vi "Pre Launch Init.vi"(11 "ZenGage v3.0 UI in":refnum<class "ZenGage v3.0 UI.lvclass">) -> (0 "error out":errorcluster, 3 "ZenGage v3.0 UI out":refnum<class "ZenGage v3.0 UI.lvclass">)   [LabVIEW 2019, in "ZenGage v3.0 UI.lvclass"]
doc: "(<B>Filename</B>: Actor Framework.lvlib:Actor.lvclass:Pre Launch Init.vi)\n\nDefines behavior that occurs after the Launch Nested Actor method is invoked but before the actor's Actor Core method begins running.\n\nBy default, this method does nothing. A descendant class may override it to define behavior."
uses:
  ZenGage v3.0 UI.lvclass
  <vilib>/vision/Image Controls.llb/IMAQ Image.ctl
  Type Definitions/User Events UI/LoadingBar_General_UI.ctl
  Type Definitions/User Events UI/Stop slave cluster.ctl
  Type Definitions/User Events UI/Optics diagnostics cluster.ctl
  Type Definitions/JSON Read/Data initialization.ctl
  Type Definitions/JSON Read/Post select init.ctl
  Type Definitions/Diagnostics/Trigger sensor.ctl
  Common/Controls/Pop-up Input.ctl
  Type Definitions/Inspection/Result Cluster.ctl
  <vilib>/ActorFramework/Actor/Actor.lvclass
  Type Definitions/JSON Read/UI JSON read cluster.ctl
  Type Definitions/General/JSONRead.ctl
  Type Definitions/Inspection/Inspection Cluster.ctl
  Type Definitions/Diagnostics/Diagnostics(Cluster).ctl
  Type Definitions/Edit tolerance settings/Rack Selection.ctl
  <vilib>/Utility/miscctls.llb/LVPoint32TypeDef.ctl
  Type Definitions/Edit tolerance settings/Edit Tolerance Input.ctl
  Type Definitions/Edit tolerance settings/Edit Tolerance Overall Cluster.ctl
  Type Definitions/Controls and Indicators/Inspection control references.ctl
  Type Definitions/Controls and Indicators/Diagnostics control referencs.ctl
  Type Definitions/Controls and Indicators/EDL control references.ctl
  Type Definitions/Controls and Indicators/Controls and Indicators Cluster.ctl
  Type Definitions/General/UI States(UI button enable disable).ctl
  Type Definitions/General/UIDataCluster.ctl
  Type Definitions/Controls and Indicators/General_Control references.ctl
  Type Definitions/General/Master sample references.ctl
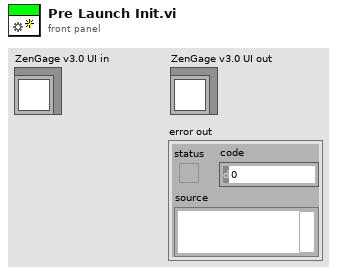
[diagram p1: front panel]
types:
  T1 = cluster{"Master sample message":string, "Part message":string}
  T2 = typedef "ZenGage v3.0 UI.lvclass/Result Cluster.ctl" = cluster{"Rack Id":u64, "Measurement Values Array ":dbl[], "Images_Array_in":T3[], "ResultPF":bool, "Production count details":cluster{"Total Count":dbl, "Total Pass":dbl, "Total Fail":dbl}, "Control Pass Fail":bool[], "ReelCount Details":cluster{"Reel Count":dbl, "Reel Pass":dbl, "Reel Fail":dbl}, "Specification Pass Fail":bool[], "SpecificationFail":bool}
  T3 = typedef "IMAQ Image.ctl" = refnum<image>
  T4 = typedef "UIDataCluster.ctl" = cluster{"JSONRead":T5, "Inspection":T7, "Diagnostics":T8, "EditToleranceSettings":T9, "ControlsIndicators":T13, "AdditionalFeatures":cluster{"Cp Cpk details":cluster{"CpCpkData":string[][], "Cp Cpk popup":refnum<vi>}, "Popup":cluster{"Restore main tab":string, "Popup data":cluster{"Loading bar data":cluster{"Open?":bool, "Display string":string}, "Pop-up":T19}}, "DynamicImageHandling":cluster{"Image update":cluster{"Rack Id":i32, "Update image":bool[]}[], "RBCIA":cluster{"Rack Id":u8, "Imaging view names":string[]}[], "ISIM":u8[], "Camera labels list":string[], "Enable DIH?":bool, "Init DIH params?":bool}, "PageHandling":cluster{"Previous State":T20, "Current state":string, "Previous control access state":string}, "Core":cluster{"Current VI Reference":refnum<vi>, "Close Panel on Exit?":bool}, "SlaveLoopData":cluster{"EnableShortKeyPress":bool, "Point32":T12}, "Chosen event reason":string, "Master sample validation":cluster{"Master sample general message":string, "Master sample part message":string}, "Fail Ignore Count Reversal":cluster{"Production ignored count":u64, "Reel ignored count":u64}}}
  T5 = typedef "ZenGage v3.0 UI.lvclass/JSONRead.ctl" = cluster{"ConfigurationFilePaths":cluster{"Default JSON Path in":path, "Rack Controller Override JSON file path in":path, "Algorithm Overrride JSON file path in ":path}, "ConfigurationVariants":cluster{"Default JSON \nVariant":variant, "Algorithm Override\nJSON Variant":variant, "Rack Controller Override\nJSON Variant":variant}, "ConfigurationCluster":T6}
  T6 = typedef "ZenGage v3.0 UI.lvclass/UI JSON read cluster.ctl" = cluster{"UIParameters":cluster{"SpecificationVersion":string, "Title":string, "NumberOfImagesToBeDisplayed":dbl, "ImageCountWindow":dbl, "FontName":string, "FontSize":dbl, "CustomerLogoFilePath":string, "ZentronLogoFilePath":string, "CompatibleSoftwareVersions":string[], "CameraLabelMapping":cluster{"CameraName":string, "ImageLabel":string}[], "ImageIndicatorLayouts":cluster{"NumberOfImageIndicators":dbl, "ImageSpecificData":cluster{"Width":dbl, "Left":dbl, "Top":dbl, "ImagePercentage":cluster{"Height":dbl, "Widthcorrection":i64, "Heightcorrection":i64, "Leftcorrection":dbl, "Topcorrection":dbl}, "StringPercentage":cluster{"Height":dbl, "Widthcorrection":i64, "Heightcorrection":dbl, "Leftcorrection":dbl, "Topcorrection":dbl}}[]}[], "SoftwareButtonLabels":cluster{"SelectLabel":string, "RunLabel":string, "PauseLabel":string, "StopLabel":string}, "DiagnosticsParameters":cluster{"CameraOpticsDiagnostics":cluster{"Label":string, "CameraLabelsList":cluster{"CameraName":string, "ImageLabel":string}[]}, "ArduinoDiagnostics":cluster{"Label":string}, "MotorDiagnostics":cluster{"Label":string}, "ReelerMotor":cluster{"Label":string}, "TowerLampDiagnostics":cluster{"Label":string}, "TriggerSensor":cluster{"Label":string, "SensorsList":cluster{"SensorName":string, "LabelName":string}[]}, "HardwareButtonDiagnostics":cluster{"Label":string}, "MasterSampleDiagnostics":cluster{"Label":string}}, "DieIdParameters":cluster{"DefaultDieId":string, "DieIdsList":string[]}, "EventReasonsList":cluster{"Pause":string[], "Stop":string[], "FailPause":string[], "Ignored":string[], "DefaultEventReason":string}, "StampingMachineIds":string[], "ErrorPopupStrings":cluster{"ErrorCode":string, "ErrorString":string}[]}}
  T7 = typedef "ZenGage v3.0 UI.lvclass/Inspection Cluster.ctl" = cluster{"Inspection After Stop":bool, "IsPaused":bool, "Camera Names":string[], "Fail Array":bool[], "Reel Number":u32, "Image details_init":cluster{"Mapped view names":string[], "Camera image map array":i32[], "Camera names":string[]}[], "LSL":string[], "USL":string[], "Max limits":cluster{"Production max":u64, "Reel max":u64}, "parts List":string[], "#Racks":u8, "MeasurementNames":string[], "Reel complete":bool, "Fail event reason list":string[]}
  T8 = typedef "ZenGage v3.0 UI.lvclass/Diagnostics(Cluster).ctl" = cluster{"Selection Done?":bool, "Diagnostics details":cluster{"Diagnostics names":cluster{"Main diagnostics":string[], "Sub diagnostics names":cluster{"Camera optics":string[], "Trigger sensor":string[]}}, "Diagnostics labels":cluster{"Main diagnostics":string[], "Sub diagnostics names":cluster{"Camera optics":string[], "Trigger sensor":string[]}}}, "DiagnosticsFeatures":cluster{"ArduinoDiagnostics":bool, "MotorDiagnostics":bool, "CameraOpticsDiagnostics":bool, "ReelerMotor":bool, "HardwareButtonDiagnostics":bool, "TriggerSensor":bool, "TowerLampDiagnostics":bool, "MasterSampleDiagnostics":bool}, "SelectedDiagnostics":string}
  T9 = typedef "ZenGage v3.0 UI.lvclass/Edit Tolerance Overall Cluster.ctl" = cluster{"Input ListBox":T10, "Saved?":bool, "IsETLSelected":bool, "IsPartSelected":bool}
  T10 = typedef "ZenGage v3.0 UI.lvclass/Edit Tolerance Input.ctl" = cluster{"Measurement Values":string[][], "Cluster of Limits":cluster{"LSL":dbl, "USL":dbl, "LCL":dbl, "UCL":dbl}, "Rack Selection":T11, "M and N Array":cluster{"M1":u64, "M2":u64, "N1":u64, "N2":u64}[], "Ticked Measurement Index":u32[], "Measurements Enabled":bool[], "Current Active Position":T12, "Current ticked measurement":dbl}
  T11 = typedef "ZenGage v3.0 UI.lvclass/Rack Selection.ctl" = enum16{"Both Racks", "Rack 2", "Rack 1"}
  T12 = typedef "LVPoint32TypeDef.ctl" = cluster{"Horizontal":i32, "Vertical":i32}
  T13 = typedef "ZenGage v3.0 UI.lvclass/Controls and Indicators Cluster.ctl" = cluster{"General":T14, "Inspection":T15, "Diagnostics":T16, "Edit Tolerance Limits":T17, "Master sample":T18}
  T14 = typedef "ZenGage v3.0 UI.lvclass/General_Control references.ctl" = cluster{"Main Tab":refnum<vi>, "Inspection SubPanel_Inspection":refnum<vi>, "Zen Logo_Inspection":refnum<vi>, "SoftwareExit":refnum<vi>, "Loading Bar VI Ref":refnum<vi>, "Right Pane Tab":refnum<vi>, "Image Reference array":refnum<vi>[], "Command tab":refnum<vi>, "Inspection subTab control ref":refnum<vi>, "SelectionCluster":cluster{"ok":refnum<vi>, "confirm":refnum<vi>, "reset":refnum<vi>, "change":refnum<vi>, "TOTAL COUNT":refnum<vi>, "REEL COUNT":refnum<vi>, "PART NAME":refnum<vi>, "VERIFIED":refnum<vi>, "OPERATOR NAME":refnum<vi>, "Select message":refnum<vi>}, "Event  Reason  List":refnum<vi>, "Event reason blink":refnum<vi>, "Event reason switching tab":refnum<vi>, "confirm_eventReason":refnum<vi>}
  T15 = typedef "ZenGage v3.0 UI.lvclass/Inspection control references.ctl" = cluster{"Inspection Status":refnum<vi>, "Run_Inspection":refnum<vi>, "Pause_Inspection":refnum<vi>, "Stop_Inspection":refnum<vi>, "Settings_Inspection":refnum<vi>, "Inspection Images VI Ref":refnum<vi>, "Pass-Fail Indicator String":refnum<vi>, "Analytics_Inspection":refnum<vi>, "Label array":refnum<vi>[], "Analytics VI\nreference":refnum<vi>, "Counts":refnum<vi>, "Cards array":refnum<vi>, "Counts array":refnum<vi>[]}
  T16 = typedef "ZenGage v3.0 UI.lvclass/Diagnostics control referencs.ctl" = cluster{"Diagnostics Tab":refnum<vi>, "Dust indicator :":refnum<vi>, "Logout_Diagnostics":refnum<vi>, "CAMERA STATUS MESSAGE":refnum<vi>, "BUZZER OFF":refnum<vi>, "PAUSE":refnum<vi>, "STOP":refnum<vi>, "RUN":refnum<vi>, "Current Diagnostics Status":refnum<vi>, "Select a diagnostics":refnum<vi>, "Diagnostics Status":refnum<vi>, "Select a sub diagnostics":refnum<vi>, "Optics img":refnum<vi>, "Diagnostics Status\nString":refnum<vi>}
  T17 = typedef "ZenGage v3.0 UI.lvclass/EDL control references.ctl" = cluster{"Tolerance Limits Listbox":refnum<vi>, "Enable Disable":refnum<vi>, "Cluster of limits":refnum<vi>, "Thresholds limits":refnum<vi>, "Update List":refnum<vi>, "Save":refnum<vi>, "Back_Edit Tolerance":refnum<vi>, "logout":refnum<vi>, "Select a part":refnum<vi>, "Bias Correction":refnum<vi>, "Linearity Correction":refnum<vi>, "Select a Rack":refnum<vi>, "ETS tab":refnum<vi>, "Factory reset":refnum<vi>, "Door\nPoka Yoke":refnum<vi>, "Fail count reverse":refnum<vi>, "ETL count error message":refnum<vi>, "ETL help string":refnum<vi>}
  T18 = typedef "Master sample references.ctl" = cluster{"Master sample message":refnum<vi>, "Master sample tab":refnum<vi>, "Next":refnum<vi>, "Repeat":refnum<vi>, "Master sample part message":refnum<vi>}
  T19 = typedef "Pop-up Input.ctl" = cluster{"Pop-up Type":enum16{"Open Logo Display", "Close Logo Display", "Open Loading Bar", "Close Loading Bar", "Open Alert Display", "Close Alert Display", "One button dialog box", "Two button dialog box", "User Authentication"}, "Title":string, "Message":string, "Button 1 Text":string, "Button 2 Text":string, "Show Close? T/F":bool, "Title Blink? T/F":bool, "Title Blink Colour":u32}
  T20 = typedef "ZenGage v3.0 UI.lvclass/UI States(UI button enable disable).ctl" = cluster{"Inspection":cluster{"Inspection States":enum16{"PreSelect", "Back _Inspection", "Analytics", "Ready To Run", "Ready To Insert", "Enable All buttons", "Disable All Buttons", "Settings", "Select", "Stop", "Pause", "Inspect"}}, "Diagnostics":cluster{"Diagnostics States":enum16{"Enable All", "Camera Optics Fail", "Loading Bar", "Camera Optics", "Motor", "Arduino", "POST Done", "POST"}}, "Edit Tolerance":cluster{"Edit Limits":enum16{"Update List"}, "Enable Disable Measurements":enum16{"Back to Edit Tolerance"}, "Page Select":enum16{"Edit Tolerance Limits", "Enable Disable Buttons"}}, "Page Select":enum16{"Edit Tolerance", "Diagnostics", "Inspection"}}
  T21 = typedef "ZenGage v3.0 UI.lvclass/Post select init.ctl" = cluster{"PartName":string, "RackId":u8, "ReInitialize":bool, "MeasurementNames":string[], "SpecValues":cluster{"LCL":dbl, "UCL":dbl, "LSL":dbl, "USL":dbl, "NominalValue":dbl}[], "CameraNames":string[]}
  T22 = typedef "ZenGage v3.0 UI.lvclass/Data initialization.ctl" = cluster{"DiagnosticsFeatures":cluster{"ArduinoDiagnostics":bool, "MotorDiagnostics":bool, "CameraOpticsDiagnostics":bool, "ReelerMotor":bool, "TowerLampDiagnostics":bool, "HardwareButtonDiagnostics":bool, "TriggerSensor":bool, "MasterSampleDiagnostics":bool}, "UserInterfaceButtonVisibilty":cluster{"Door Poka Yoke":bool, "DynamicImageHandlingEnable":bool, "FailCountDisplayButtonVisible":bool, "FailCountReversalButtonVisible":bool}, "Analytics enabled":bool, "Parts List":cluster{"Part name":string, "NumberOfRacks":u8}[]}
  T23 = typedef "ZenGage v3.0 UI.lvclass/Trigger sensor.ctl" = cluster{"Image":T3[], "CaptureCount":u64}
  T24 = typedef "ZenGage v3.0 UI.lvclass/Optics diagnostics cluster.ctl" = cluster{"DustPercentage":dbl, "Pass":bool, "FinalImage":T3}
  T25 = typedef "ZenGage v3.0 UI.lvclass/LoadingBar_General_UI.ctl" = cluster{"Open?":bool, "Loading string?":string}
  T26 = typedef "ZenGage v3.0 UI.lvclass/Stop slave cluster.ctl" = cluster{"Stop UI?":bool}
  T27 = typedef "ZenGage v3.0 UI.lvclass/UserEvents_UI.ctl" = cluster{"LoadingBar_General_UI":refnum<user-event>, "OpticsDiagnostics_UI":refnum<user-event>, "DisplayResult_UI":refnum<user-event>, "DisplayPopup_UI":refnum<user-event>, "DisplayProcessCapabilityPopup_UI":refnum<user-event>, "ButtonPress_UI":refnum<user-event>, "GetAnalyticsVI_UI":refnum<user-event>, "SystemInfo_UI":refnum<user-event>, "PartInfo_UI":refnum<user-event>, "TriggerSensorDiagnostics_UI":refnum<user-event>, "AskEventReason_UI":refnum<user-event>, "Display CpCpk data_UI":refnum<user-event>, "MasterSampleMessageUpdate_UI":refnum<user-event>}
  T28 = cluster{"Stop slave user event_UI":refnum<user-event>, "Enable shortkey":refnum<user-event>, "SendClusterData":refnum<user-event>, "SendClusterData to MainLoop":refnum<user-event>}
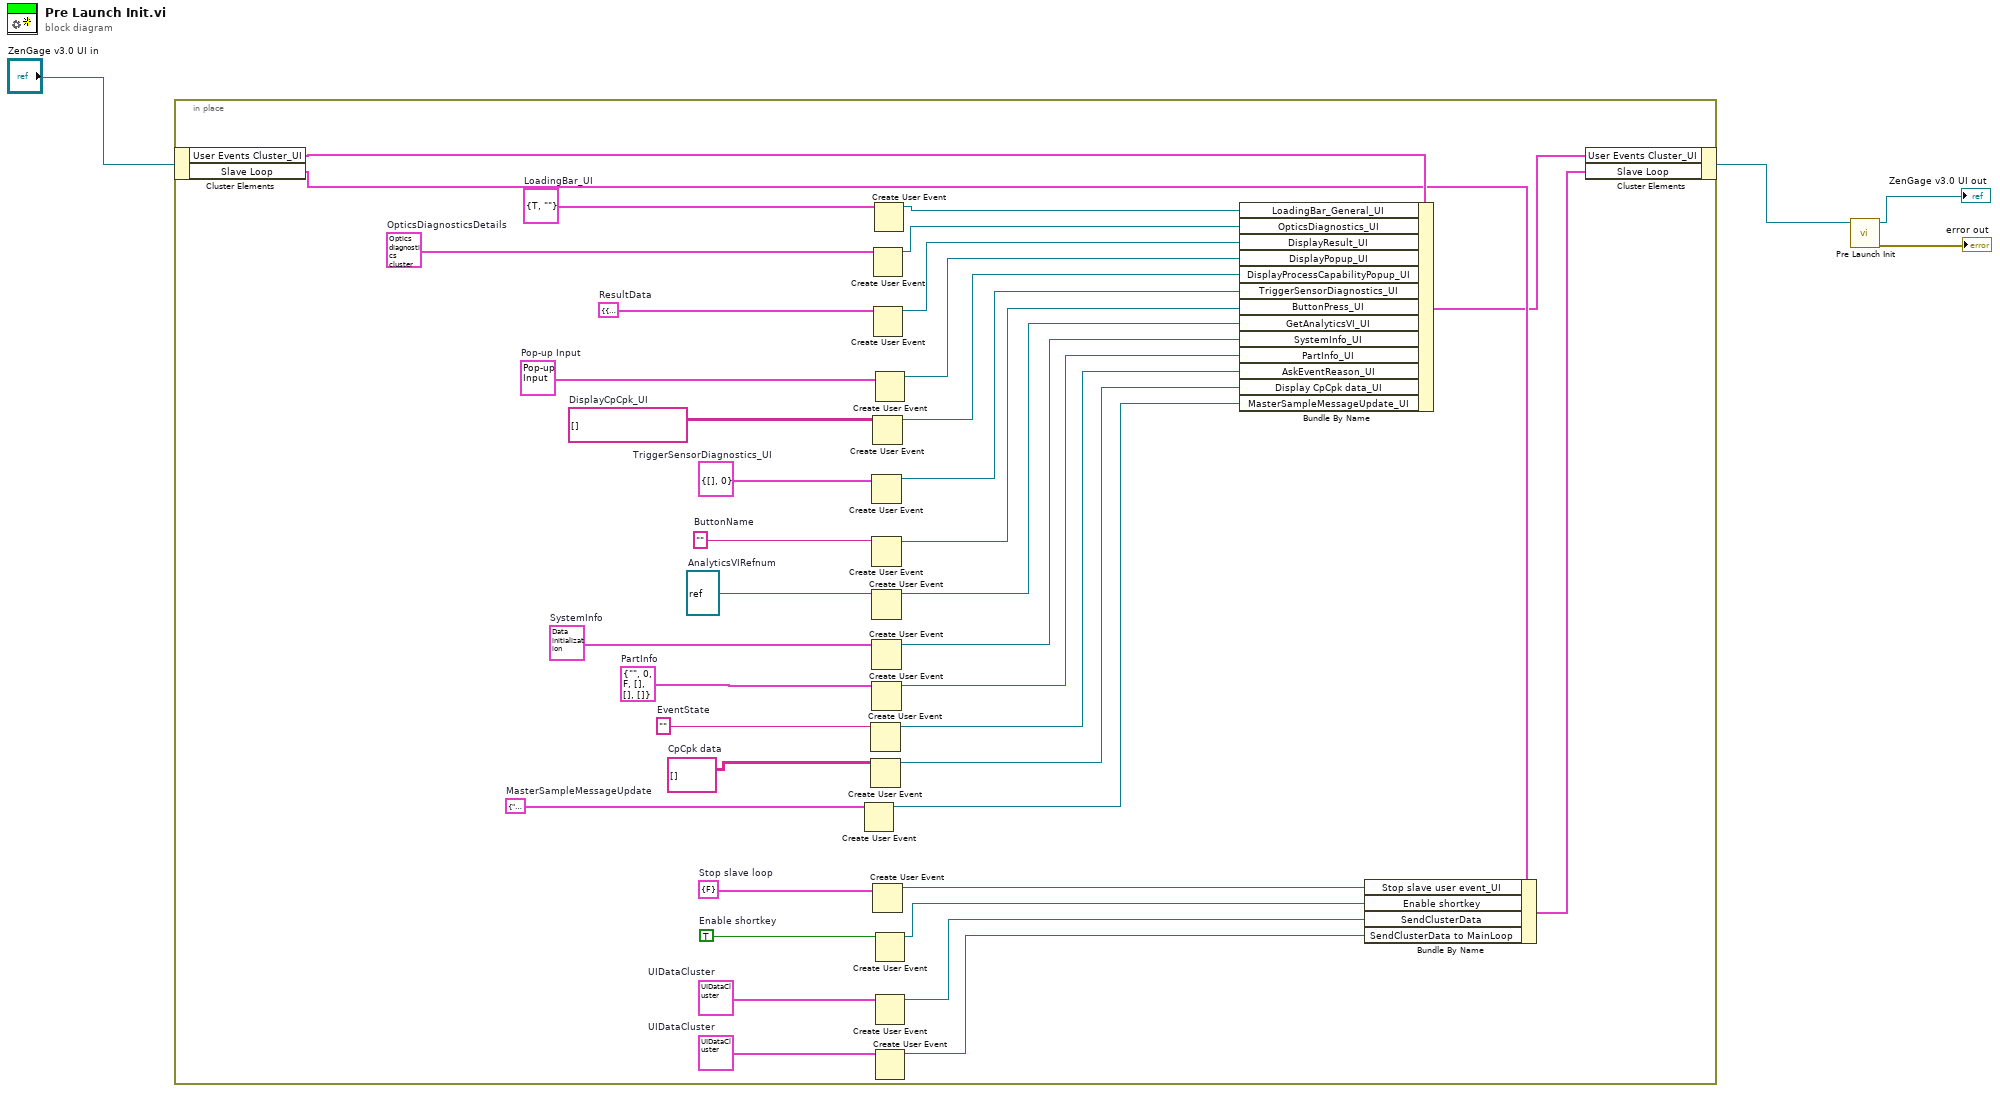
[diagram p0: block diagram]
diagram:
  n1 = in-place {
    w6 = T1 {"Master sample message"="", "Part message"=""}  # MasterSampleMessageUpdate
    w7 = cluster{"Result Cluster 2":T2} {"Result Cluster 2"={"Rack Id"=0, "Measurement Values Array "=[], "Images_Array_in"=[], "ResultPF"=FALSE, "Production count details"={"Total Count"=0.0, "Total Pass"=0.0, "Total Fail"=0.0}, "Control Pass Fail"=[], "ReelCount Details"={"Reel Count"=0.0, "Reel Pass"=0.0, "Reel Fail"=0.0}, "Specification Pass Fail"=[], "SpecificationFail"=FALSE}}  # ResultData
    w9 = string[][] []  # CpCpk data
    w11 = T4 {"JSONRead"={"ConfigurationFilePaths"={"Default JSON Path in"=path "", "Rack Controller Override JSON file path in"=path "", "Algorithm Overrride JSON file path in "=path ""}, "ConfigurationVariants"={"Default JSON \nVariant"=variant, "Algorithm Override\nJSON Variant"=variant, "Rack Controller Override\nJSON Variant"=variant}, "ConfigurationCluster"={"UIParameters"={"SpecificationVersion"="", "Title"="", "NumberOfImagesToBeDisplayed"=0.0, "ImageCountWindow"=0.0, "FontName"="", "FontSize"=0.0, "CustomerLogoFilePath"="", "ZentronLogoFilePath"="", "CompatibleSoftwareVersions"=[], "CameraLabelMapping"=[], "ImageIndicatorLayouts"=[], "SoftwareButtonLabels"={"SelectLabel"="", "RunLabel"="", "PauseLabel"="", "StopLabel"=""}, "DiagnosticsParameters"={"CameraOpticsDiagnostics"={"Label"="", "CameraLabelsList"=[]}, "ArduinoDiagnostics"={"Label"=""}, "MotorDiagnostics"={"Label"=""}, "ReelerMotor"={"Label"=""}, "TowerLampDiagnostics"={"Label"=""}, "TriggerSensor"={"Label"="", "SensorsList"=[]}, "HardwareButtonDiagnostics"={"Label"=""}, "MasterSampleDiagnostics"={"Label"=""}}, "DieIdParameters"={"DefaultDieId"="", "DieIdsList"=[]}, "EventReasonsList"={"Pause"=[], "Stop"=[], "FailPause"=[], "Ignored"=[], "DefaultEventReason"=""}, "StampingMachineIds"=[], "ErrorPopupStrings"=[]}}}, "Inspection"={"Inspection After Stop"=FALSE, "IsPaused"=FALSE, "Camera Names"=[], "Fail Array"=[], "Reel Number"=0, "Image details_init"=[], "LSL"=[], "USL"=[], "Max limits"={"Production max"=0, "Reel max"=0}, "parts List"=[], "#Racks"=0, "MeasurementNames"=[], "Reel complete"=FALSE, "Fail event reason list"=[]}, "Diagnostics"={"Selection Done?"=FALSE, "Diagnostics details"={"Diagnostics names"={"Main diagnostics"=[], "Sub diagnostics names"={"Camera optics"=[], "Trigger sensor"=[]}}, "Diagnostics labels"={"Main diagnostics"=[], "Sub diagnostics names"={"Camera optics"=[], "Trigger sensor"=[]}}}, "DiagnosticsFeatures"={"ArduinoDiagnostics"=FALSE, "MotorDiagnostics"=FALSE, "CameraOpticsDiagnostics"=FALSE, "ReelerMotor"=FALSE, "HardwareButtonDiagnostics"=FALSE, "TriggerSensor"=FALSE, "TowerLampDiagnostics"=FALSE, "MasterSampleDiagnostics"=FALSE}, "SelectedDiagnostics"=""}, "EditToleranceSettings"={"Input ListBox"={"Measurement Values"=[], "Cluster of Limits"={"LSL"=0.0, "USL"=0.0, "LCL"=0.0, "UCL"=0.0}, "Rack Selection"=enum."Both Racks", "M and N Array"=[], "Ticked Measurement Index"=[], "Measurements Enabled"=[], "Current Active Position"={"Horizontal"=0, "Vertical"=0}, "Current ticked measurement"=0.0}, "Saved?"=FALSE, "IsETLSelected"=FALSE, "IsPartSelected"=FALSE}, "ControlsIndicators"={"General"={"Main Tab"=refnum, "Inspection SubPanel_Inspection"=refnum, "Zen Logo_Inspection"=refnum, "SoftwareExit"=refnum, "Loading Bar VI Ref"=refnum, "Right Pane Tab"=refnum, "Image Reference array"=[], "Command tab"=refnum, "Inspection subTab control ref"=refnum, "SelectionCluster"={"ok"=refnum, "confirm"=refnum, "reset"=refnum, "change"=refnum, "TOTAL COUNT"=refnum, "REEL COUNT"=refnum, "PART NAME"=refnum, "VERIFIED"=refnum, "OPERATOR NAME"=refnum, "Select message"=refnum}, "Event  Reason  List"=refnum, "Event reason blink"=refnum, "Event reason switching tab"=refnum, "confirm_eventReason"=refnum}, "Inspection"={"Inspection Status"=refnum, "Run_Inspection"=refnum, "Pause_Inspection"=refnum, "Stop_Inspection"=refnum, "Settings_Inspection"=refnum, "Inspection Images VI Ref"=refnum, "Pass-Fail Indicator String"=refnum, "Analytics_Inspection"=refnum, "Label array"=[], "Analytics VI\nreference"=refnum, "Counts"=refnum, "Cards array"=refnum, "Counts array"=[]}, "Diagnostics"={"Diagnostics Tab"=refnum, "Dust indicator :"=refnum, "Logout_Diagnostics"=refnum, "CAMERA STATUS MESSAGE"=refnum, "BUZZER OFF"=refnum, "PAUSE"=refnum, "STOP"=refnum, "RUN"=refnum, "Current Diagnostics Status"=refnum, "Select a diagnostics"=refnum, "Diagnostics Status"=refnum, "Select a sub diagnostics"=refnum, "Optics img"=refnum, "Diagnostics Status\nString"=refnum}, "Edit Tolerance Limits"={"Tolerance Limits Listbox"=refnum, "Enable Disable"=refnum, "Cluster of limits"=refnum, "Thresholds limits"=refnum, "Update List"=refnum, "Save"=refnum, "Back_Edit Tolerance"=refnum, "logout"=refnum, "Select a part"=refnum, "Bias Correction"=refnum, "Linearity Correction"=refnum, "Select a Rack"=refnum, "ETS tab"=refnum, "Factory reset"=refnum, "Door\nPoka Yoke"=refnum, "Fail count reverse"=refnum, "ETL count error message"=refnum, "ETL help string"=refnum}, "Master sample"={"Master sample message"=refnum, "Master sample tab"=refnum, "Next"=refnum, "Repeat"=refnum, "Master sample part message"=refnum}}, "AdditionalFeatures"={"Cp Cpk details"={"CpCpkData"=[], "Cp Cpk popup"=refnum}, "Popup"={"Restore main tab"="", "Popup data"={"Loading bar data"={"Open?"=FALSE, "Display string"=""}, "Pop-up"={"Pop-up Type"=enum."Open Logo Display", "Title"="", "Message"="", "Button 1 Text"="", "Button 2 Text"="", "Show Close? T/F"=FALSE, "Title Blink? T/F"=FALSE, "Title Blink Colour"=0}}}, "DynamicImageHandling"={"Image update"=[], "RBCIA"=[], "ISIM"=[], "Camera labels list"=[], "Enable DIH?"=FALSE, "Init DIH params?"=FALSE}, "PageHandling"={"Previous State"={"Inspection"={"Inspection States"=enum."PreSelect"}, "Diagnostics"={"Diagnostics States"=enum."Enable All"}, "Edit Tolerance"={"Edit Limits"=enum."Update List", "Enable Disable Measurements"=enum."Back to Edit Tolerance", "Page Select"=enum."Edit Tolerance Limits"}, "Page Select"=enum."Edit Tolerance"}, "Current state"="", "Previous control access state"=""}, "Core"={"Current VI Reference"=refnum, "Close Panel on Exit?"=FALSE}, "SlaveLoopData"={"EnableShortKeyPress"=FALSE, "Point32"={"Horizontal"=0, "Vertical"=0}}, "Chosen event reason"="", "Master sample validation"={"Master sample general message"="", "Master sample part message"=""}, "Fail Ignore Count Reversal"={"Production ignored count"=0, "Reel ignored count"=0}}}  # UIDataCluster
    w14 = T4 {"JSONRead"={"ConfigurationFilePaths"={"Default JSON Path in"=path "", "Rack Controller Override JSON file path in"=path "", "Algorithm Overrride JSON file path in "=path ""}, "ConfigurationVariants"={"Default JSON \nVariant"=variant, "Algorithm Override\nJSON Variant"=variant, "Rack Controller Override\nJSON Variant"=variant}, "ConfigurationCluster"={"UIParameters"={"SpecificationVersion"="", "Title"="", "NumberOfImagesToBeDisplayed"=0.0, "ImageCountWindow"=0.0, "FontName"="", "FontSize"=0.0, "CustomerLogoFilePath"="", "ZentronLogoFilePath"="", "CompatibleSoftwareVersions"=[], "CameraLabelMapping"=[], "ImageIndicatorLayouts"=[], "SoftwareButtonLabels"={"SelectLabel"="", "RunLabel"="", "PauseLabel"="", "StopLabel"=""}, "DiagnosticsParameters"={"CameraOpticsDiagnostics"={"Label"="", "CameraLabelsList"=[]}, "ArduinoDiagnostics"={"Label"=""}, "MotorDiagnostics"={"Label"=""}, "ReelerMotor"={"Label"=""}, "TowerLampDiagnostics"={"Label"=""}, "TriggerSensor"={"Label"="", "SensorsList"=[]}, "HardwareButtonDiagnostics"={"Label"=""}, "MasterSampleDiagnostics"={"Label"=""}}, "DieIdParameters"={"DefaultDieId"="", "DieIdsList"=[]}, "EventReasonsList"={"Pause"=[], "Stop"=[], "FailPause"=[], "Ignored"=[], "DefaultEventReason"=""}, "StampingMachineIds"=[], "ErrorPopupStrings"=[]}}}, "Inspection"={"Inspection After Stop"=FALSE, "IsPaused"=FALSE, "Camera Names"=[], "Fail Array"=[], "Reel Number"=0, "Image details_init"=[], "LSL"=[], "USL"=[], "Max limits"={"Production max"=0, "Reel max"=0}, "parts List"=[], "#Racks"=0, "MeasurementNames"=[], "Reel complete"=FALSE, "Fail event reason list"=[]}, "Diagnostics"={"Selection Done?"=FALSE, "Diagnostics details"={"Diagnostics names"={"Main diagnostics"=[], "Sub diagnostics names"={"Camera optics"=[], "Trigger sensor"=[]}}, "Diagnostics labels"={"Main diagnostics"=[], "Sub diagnostics names"={"Camera optics"=[], "Trigger sensor"=[]}}}, "DiagnosticsFeatures"={"ArduinoDiagnostics"=FALSE, "MotorDiagnostics"=FALSE, "CameraOpticsDiagnostics"=FALSE, "ReelerMotor"=FALSE, "HardwareButtonDiagnostics"=FALSE, "TriggerSensor"=FALSE, "TowerLampDiagnostics"=FALSE, "MasterSampleDiagnostics"=FALSE}, "SelectedDiagnostics"=""}, "EditToleranceSettings"={"Input ListBox"={"Measurement Values"=[], "Cluster of Limits"={"LSL"=0.0, "USL"=0.0, "LCL"=0.0, "UCL"=0.0}, "Rack Selection"=enum."Both Racks", "M and N Array"=[], "Ticked Measurement Index"=[], "Measurements Enabled"=[], "Current Active Position"={"Horizontal"=0, "Vertical"=0}, "Current ticked measurement"=0.0}, "Saved?"=FALSE, "IsETLSelected"=FALSE, "IsPartSelected"=FALSE}, "ControlsIndicators"={"General"={"Main Tab"=refnum, "Inspection SubPanel_Inspection"=refnum, "Zen Logo_Inspection"=refnum, "SoftwareExit"=refnum, "Loading Bar VI Ref"=refnum, "Right Pane Tab"=refnum, "Image Reference array"=[], "Command tab"=refnum, "Inspection subTab control ref"=refnum, "SelectionCluster"={"ok"=refnum, "confirm"=refnum, "reset"=refnum, "change"=refnum, "TOTAL COUNT"=refnum, "REEL COUNT"=refnum, "PART NAME"=refnum, "VERIFIED"=refnum, "OPERATOR NAME"=refnum, "Select message"=refnum}, "Event  Reason  List"=refnum, "Event reason blink"=refnum, "Event reason switching tab"=refnum, "confirm_eventReason"=refnum}, "Inspection"={"Inspection Status"=refnum, "Run_Inspection"=refnum, "Pause_Inspection"=refnum, "Stop_Inspection"=refnum, "Settings_Inspection"=refnum, "Inspection Images VI Ref"=refnum, "Pass-Fail Indicator String"=refnum, "Analytics_Inspection"=refnum, "Label array"=[], "Analytics VI\nreference"=refnum, "Counts"=refnum, "Cards array"=refnum, "Counts array"=[]}, "Diagnostics"={"Diagnostics Tab"=refnum, "Dust indicator :"=refnum, "Logout_Diagnostics"=refnum, "CAMERA STATUS MESSAGE"=refnum, "BUZZER OFF"=refnum, "PAUSE"=refnum, "STOP"=refnum, "RUN"=refnum, "Current Diagnostics Status"=refnum, "Select a diagnostics"=refnum, "Diagnostics Status"=refnum, "Select a sub diagnostics"=refnum, "Optics img"=refnum, "Diagnostics Status\nString"=refnum}, "Edit Tolerance Limits"={"Tolerance Limits Listbox"=refnum, "Enable Disable"=refnum, "Cluster of limits"=refnum, "Thresholds limits"=refnum, "Update List"=refnum, "Save"=refnum, "Back_Edit Tolerance"=refnum, "logout"=refnum, "Select a part"=refnum, "Bias Correction"=refnum, "Linearity Correction"=refnum, "Select a Rack"=refnum, "ETS tab"=refnum, "Factory reset"=refnum, "Door\nPoka Yoke"=refnum, "Fail count reverse"=refnum, "ETL count error message"=refnum, "ETL help string"=refnum}, "Master sample"={"Master sample message"=refnum, "Master sample tab"=refnum, "Next"=refnum, "Repeat"=refnum, "Master sample part message"=refnum}}, "AdditionalFeatures"={"Cp Cpk details"={"CpCpkData"=[], "Cp Cpk popup"=refnum}, "Popup"={"Restore main tab"="", "Popup data"={"Loading bar data"={"Open?"=FALSE, "Display string"=""}, "Pop-up"={"Pop-up Type"=enum."Open Logo Display", "Title"="", "Message"="", "Button 1 Text"="", "Button 2 Text"="", "Show Close? T/F"=FALSE, "Title Blink? T/F"=FALSE, "Title Blink Colour"=0}}}, "DynamicImageHandling"={"Image update"=[], "RBCIA"=[], "ISIM"=[], "Camera labels list"=[], "Enable DIH?"=FALSE, "Init DIH params?"=FALSE}, "PageHandling"={"Previous State"={"Inspection"={"Inspection States"=enum."PreSelect"}, "Diagnostics"={"Diagnostics States"=enum."Enable All"}, "Edit Tolerance"={"Edit Limits"=enum."Update List", "Enable Disable Measurements"=enum."Back to Edit Tolerance", "Page Select"=enum."Edit Tolerance Limits"}, "Page Select"=enum."Edit Tolerance"}, "Current state"="", "Previous control access state"=""}, "Core"={"Current VI Reference"=refnum, "Close Panel on Exit?"=FALSE}, "SlaveLoopData"={"EnableShortKeyPress"=FALSE, "Point32"={"Horizontal"=0, "Vertical"=0}}, "Chosen event reason"="", "Master sample validation"={"Master sample general message"="", "Master sample part message"=""}, "Fail Ignore Count Reversal"={"Production ignored count"=0, "Reel ignored count"=0}}}  # UIDataCluster
    w21 = TRUE  # Enable shortkey
    w30 = ""  # EventState
    w35 = T21 {"PartName"="", "RackId"=0, "ReInitialize"=FALSE, "MeasurementNames"=[], "SpecValues"=[], "CameraNames"=[]}  # PartInfo
    w36 = T22 {"DiagnosticsFeatures"={"ArduinoDiagnostics"=FALSE, "MotorDiagnostics"=FALSE, "CameraOpticsDiagnostics"=FALSE, "ReelerMotor"=FALSE, "TowerLampDiagnostics"=FALSE, "HardwareButtonDiagnostics"=FALSE, "TriggerSensor"=FALSE, "MasterSampleDiagnostics"=FALSE}, "UserInterfaceButtonVisibilty"={"Door Poka Yoke"=FALSE, "DynamicImageHandlingEnable"=FALSE, "FailCountDisplayButtonVisible"=FALSE, "FailCountReversalButtonVisible"=FALSE}, "Analytics enabled"=FALSE, "Parts List"=[]}  # SystemInfo
    w31 = refnum<vi> refnum  # AnalyticsVIRefnum
    w32 = string[][] []  # DisplayCpCpk_UI
    w33 = T19 {"Pop-up Type"=enum."Open Logo Display", "Title"="", "Message"="", "Button 1 Text"="", "Button 2 Text"="", "Show Close? T/F"=FALSE, "Title Blink? T/F"=FALSE, "Title Blink Colour"=0}  # Pop-up Input
    w34 = T23 {"Image"=[], "CaptureCount"=0}  # TriggerSensorDiagnostics_UI
    w37 = T24 {"DustPercentage"=90.0, "Pass"=FALSE, "FinalImage"=refnum}  # OpticsDiagnosticsDetails
    w42 = T25 {"Open?"=TRUE, "Loading string?"=""}  # LoadingBar_UI
    w38 = ""  # ButtonName
    w40 = T26 {"Stop UI?"=FALSE}  # Stop slave loop
    n2 = in-place-cluster #1("ZenGage v3.0 UI in") -> ("User Events Cluster_UI"=w18:T27, "Slave Loop"=w17:T28)
    n3 = Create User Event(user event datatype=w6) -> (user event=w5:refnum<user-event>)  [unwired: 1 in, 1 out]
    n4 = Create User Event(user event datatype=w30) -> (user event=w22:refnum<user-event>)  [unwired: 1 in, 1 out]
    n5 = Create User Event(user event datatype=w9) -> (user event=w8:refnum<user-event>)  [unwired: 1 in, 1 out]
    n6 = Create User Event(user event datatype=w34) -> (user event=w26:refnum<user-event>)  [unwired: 1 in, 1 out]
    n7 = Create User Event(user event datatype=w38) -> (user event=w12:refnum<user-event>)  [unwired: 1 in, 1 out]
    n8 = Create User Event(user event datatype=w31) -> (user event=w25:refnum<user-event>)  [unwired: 1 in, 1 out]
    n9 = Create User Event(user event datatype=w36) -> (user event=w24:refnum<user-event>)  [unwired: 1 in, 1 out]
    n10 = Create User Event(user event datatype=w35) -> (user event=w23:refnum<user-event>)  [unwired: 1 in, 1 out]
    n11 = Create User Event(user event datatype=w32) -> (user event=w27:refnum<user-event>)  [unwired: 1 in, 1 out]
    n12 = Create User Event(user event datatype=w40) -> (user event=w39:refnum<user-event>)  [unwired: 1 in, 1 out]
    n13 = Create User Event(user event datatype=w37) -> (user event=w29:refnum<user-event>)  [unwired: 1 in, 1 out]
    n14 = Create User Event(user event datatype=w7) -> (user event=w19:refnum<user-event>)  [unwired: 1 in, 1 out]
    n15 = Create User Event(user event datatype=w42) -> (user event=w41:refnum<user-event>)  [unwired: 1 in, 1 out]
    n16 = Create User Event(user event datatype=w33) -> (user event=w28:refnum<user-event>)  [unwired: 1 in, 1 out]
    n17 = Create User Event(user event datatype=w21) -> (user event=w20:refnum<user-event>)  [unwired: 1 in, 1 out]
    n18 = Create User Event(user event datatype=w14) -> (user event=w13:refnum<user-event>)  [unwired: 1 in, 1 out]
    n19 = Create User Event(user event datatype=w11) -> (user event=w10:refnum<user-event>)  [unwired: 1 in, 1 out]
    n20 = Bundle By Name(cluster=w18, "LoadingBar_General_UI"=w41, "OpticsDiagnostics_UI"=w29, "DisplayResult_UI"=w19, "DisplayPopup_UI"=w28, "DisplayProcessCapabilityPopup_UI"=w27, "TriggerSensorDiagnostics_UI"=w26, "ButtonPress_UI"=w12, "GetAnalyticsVI_UI"=w25, "SystemInfo_UI"=w24, "PartInfo_UI"=w23, "AskEventReason_UI"=w22, "Display CpCpk data_UI"=w8, "MasterSampleMessageUpdate_UI"=w5) -> (w16:T27)
    n21 = Bundle By Name(cluster=w17, "Stop slave user event_UI"=w39, "Enable shortkey"=w20, "SendClusterData"=w13, "SendClusterData to MainLoop"=w10) -> (w15:T28)
    n22 = in-place-cluster #1("User Events Cluster_UI"=w16, "Slave Loop"=w15) -> (w1:refnum<class "ZenGage v3.0 UI.lvclass">)
  }
  n23 = call-parent "Pre Launch Init.vi"("Actor in"=w1) -> ("error out"=→"error out":errorcluster, "Actor out"=→"ZenGage v3.0 UI out":refnum<class "ZenGage v3.0 UI.lvclass">)  [unwired: 9 in]
